vi "test3.vi"() -> ()   [LabVIEW 2020]
uses:
  <vilib>/Platform/TimedLoop/XDataNode/timing_clust.ctl
  <vilib>/Platform/TimedLoop/XDataNode/nitl_modes.ctl
  <vilib>/Platform/TimedLoop/XDataNode/wakeup.ctl
  37583fcc-cec8-480d-a6d0-1da09da3d0dd.vi
  <vilib>/platform/TimedLoop/XDataNode/XDataNode.xnode
  <vilib>/Platform/TimedLoop/XDataNode/XDNodeRunTimeDep.lvlib
panel:
  out "Tank":dbl(slide) scale=0.0..1.0
  out "Current XY":cluster{"X":dbl, "Y":dbl}
  out "XY Graph":cluster{dbl[], dbl[]}[](graph)
  out "Move Time":u32
  out "Distance":dbl
  out "Start Time":u32
  out "Start XY":cluster{"X":dbl, "Y":dbl}
  out "Target XY":cluster{"X":dbl, "Y":dbl}
  out "Stopped":bool
  in  "Stop":bool
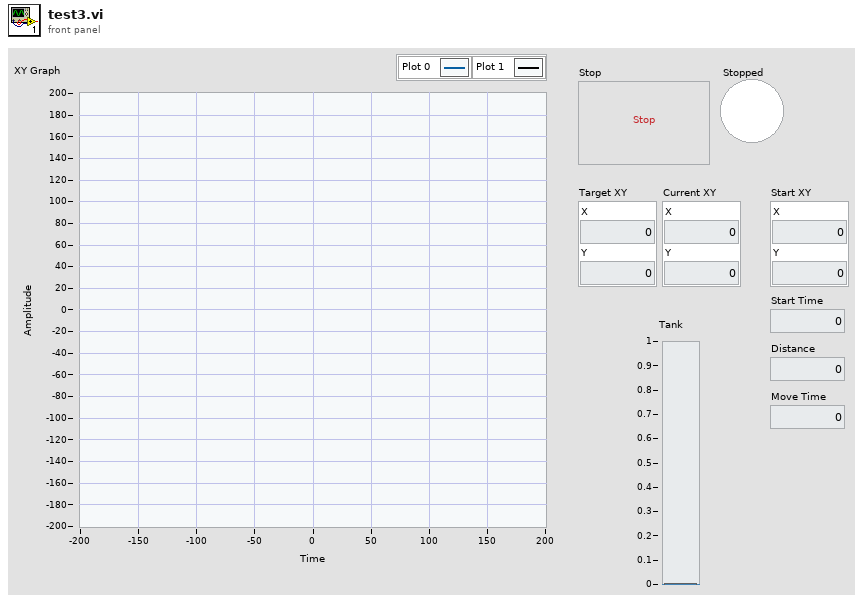
[diagram p1: front panel]
types:
  T1 = typedef "XDNodeRunTimeDep.lvlib/timing_clust.ctl" = cluster{"Expected End [f-1]":u64, "Actual End [f-1]":u64, "Finished Late? [f-1]":bool, "Expected End [i-1]":u64, "Actual End [i-1]":u64, "Finished Late? [i-1]":bool, "Expected Start [i]":u64, "Actual Start [i]":u64, "Expected Start [f]":u64, "Actual Start [f]":u64, "Source Name":string, "Structure Name":string, "Period":i64, "Deadline":i64, "Offset":i64, "Start":i64, "Priority":i32, "Timeout":i32, "Mode":T2, "Wakeup Reason":T3, "Error":errorcluster, "Source Type":string, "Secondary Source Type":string, "Global End Time":u64, "Global Start Time":u64, "Frame Duration":u64, "Iteration Duration":u64, "Assigned CPU":i32, "I/O Scan Engine Mode":u32}
  T2 = typedef "XDNodeRunTimeDep.lvlib/nitl_modes.ctl" = enum32{"No Change", "Process missed periods, maintain original phase", "Discard missed periods, maintain original phase", "Process missed periods, ignore original phase", "Discard missed periods, ignore original phase"}
  T3 = typedef "XDNodeRunTimeDep.lvlib/wakeup.ctl" = enum32{"Normal", "Aborted", "Asynchronous wakeup", "Timing source error", "Timed loop error", "Timeout"}
  T4 = typedef "LVPoint32TypeDef.ctl" = cluster{"Horizontal":i32, "Vertical":i32}
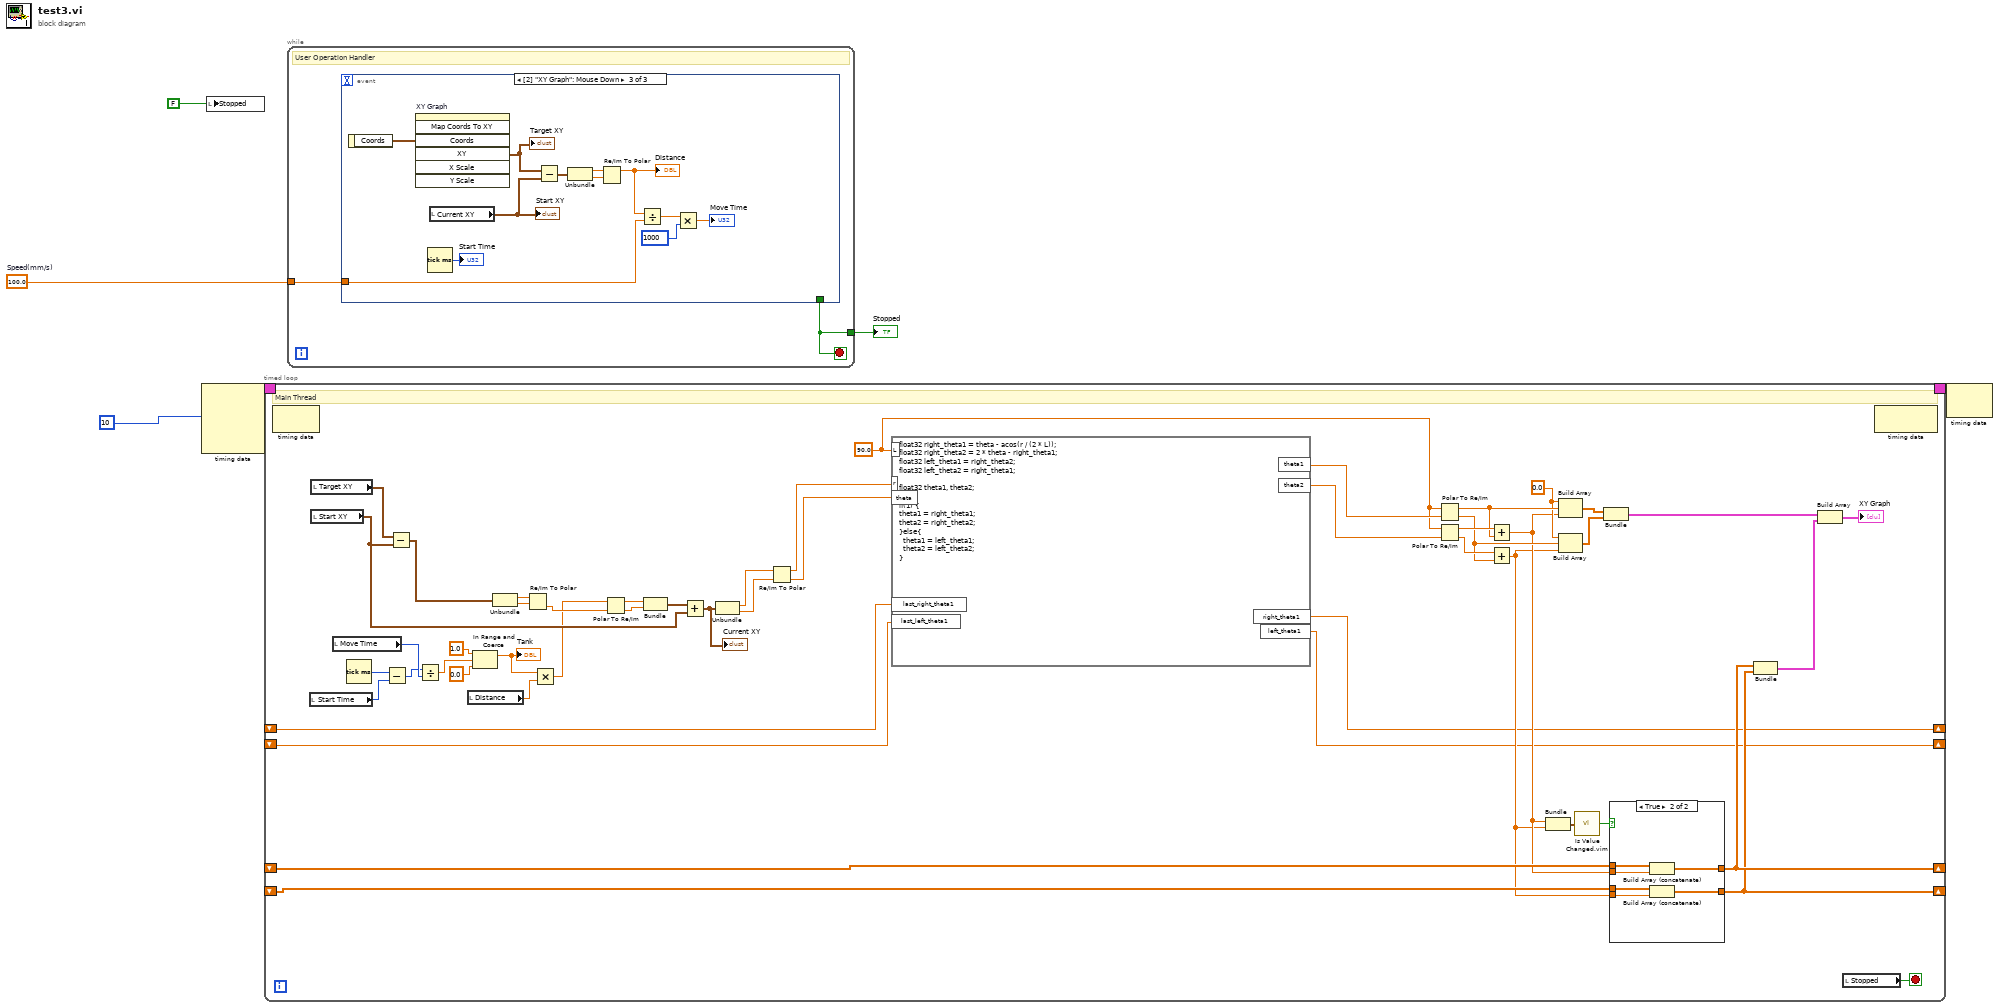
[diagram p0: block diagram]
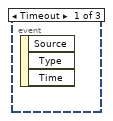
[diagram p3: hidden frame]
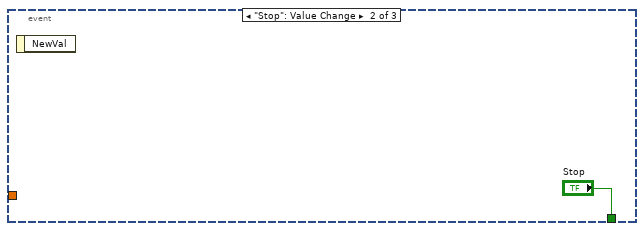
[diagram p4: hidden frame]
diagram:
  w1 = 100.0  # Speed(mm/s)
  n1 = node-c288(i64 10 ("Period")) -> (w6:T1)  [unwired: 3 in]
  n2 = local write "Stopped"(FALSE ("Stopped")) -> ()
  n3 = timed-loop {
    timing: w6 -> [_]
    timing-out: [_] -> w5
    shift-right: [w19] -> _
    shift-left: _ -> [w26]
    shift-right: [w18] -> _
    shift-left: _ -> [w25]
    shift-right: [w9] -> _
    shift-left: _ -> [w8]
    shift-right: [w10] -> _
    shift-left: _ -> [w7]
    stop <- w56 stop-if-true
    w31 = 0.0 ("element")
    w28 = 90.0 ("input variable")
    # "Main Thread"
    n4 = node-c288() -> ()  [unwired: 1 in, 1 out]
    n5 = local read "Start Time"() -> (w54:u32)
    n6 = local read "Target XY"() -> (w53:cluster{"X":dbl, "Y":dbl})
    n7 = local read "Start XY"() -> (w44:cluster{"X":dbl, "Y":dbl})
    n8 = local read "Move Time"() -> (w40:u32)
    n9 = Tick Count (ms)() -> (millisecond timer value=w55:u32)
    n10 = Subtract(x=w55, y=w54) -> (x-y=w15:u32)
    n11 = Subtract(x=w53, y=w44) -> (x-y=w51:cluster{"X":dbl, "Y":dbl})
    n12 = Divide(x=w15, y=w40) -> (x/y=w14:dbl)
    n13 = local read "Distance"() -> (w52:dbl)
    n14 = In Range and Coerce(upper limit=1.0 ("lower limit"), x=w14, lower limit=0.0) -> (coerced(x)=w11:dbl)  [unwired: 1 out]
    "Tank" <- w11
    n15 = Unbundle(w51) -> ("X"=w50:dbl, "Y"=w49:dbl)
    n16 = Re/Im To Polar(2:w49, 3:w50) -> (0:w48:dbl)  [unwired: 1 out]
    n17 = Multiply(x=w11, y=w52) -> (x*y=w39:dbl)
    n18 = Polar To Re/Im(2:w48, 3:w39) -> (0:w46:dbl, 1:w47:dbl)
    n19 = Bundle(w47, w46) -> (w45:cluster{dbl, dbl})  [unwired: 1 in]
    n20 = Add(x=w45, y=w44) -> (x+y=w27:cluster{dbl, dbl})
    "Current XY" <- w27
    n21 = Unbundle(w27) -> (w43:dbl, w42:dbl)
    n22 = Re/Im To Polar(2:w42, 3:w43) -> (0:w41:dbl, 1:w38:dbl)
    n23 = formula code="float32 right_theta1 = theta - acos(r / (2 * L));\nfloat32 right_theta2 = 2 * theta - right_theta1;\nfloat32 left_theta1 = right_theta2;\nfloat32 left_theta2 = right_theta1;\n\nfloat32 theta1, theta2;\n\nif(1) {\ntheta1 = right_theta1;\ntheta2 = right_theta2;\n}else{\n  theta1 = left_theta1;\n  theta2 = left_theta2;\n}"("r"=w38, "theta"=w41, "L"=w28, "last_right_theta1"=w8, "last_left_theta1"=w7) -> ("theta1"=w30:sgl, "theta2"=w29:sgl, "right_theta1"=w9:sgl, "left_theta1"=w10:sgl)
    n24 = Polar To Re/Im(2:w30, 3:w28) -> (0:w34:dbl, 1:w35:dbl)
    n25 = Polar To Re/Im(2:w29, 3:w28) -> (0:w36:dbl, 1:w37:dbl)
    n26 = Add(x=w37, y=w35) -> (x+y=w24:dbl)
    n27 = Add(x=w36, y=w34) -> (x+y=w23:dbl)
    n28 = Bundle(w24, w23) -> (w22:cluster{dbl, dbl})  [unwired: 1 in]
    n29 = Build Array(w31, w35, w24) -> (w33:dbl[])
    n30 = Build Array(w31, w34, w23) -> (w32:dbl[])
    n31 = call "Is Value Changed.vim"("value"=w22) -> ("changed or first call?"=w21:bool)
    n32 = Bundle(w33, w32) -> (w20:cluster{dbl[], dbl[]})  [unwired: 1 in]
    n33 = case shown="True" w21 {
      tunnel: w24 -> [_ w64]
      tunnel: w23 -> [_ w63]
      tunnel: [w58 w62] -> w19
      tunnel: [w57 w61] -> w18
      tunnel: w26 -> [w58 w60]
      tunnel: w25 -> [w57 w59]
      frame False {
      }
      frame True {
        n34 = Build Array (concatenate)(w60, w64) -> (w62:dbl[])
        n35 = Build Array (concatenate)(w59, w63) -> (w61:dbl[])
      }
    }
    n36 = Bundle(w19, w18) -> (w17:cluster{dbl[], dbl[]})  [unwired: 1 in]
    n37 = Build Array(w20, w17) -> (→"XY Graph":cluster{dbl[], dbl[]}[])
    n38 = local read "Stopped"() -> (w56:bool)
    n39 = node-c288() -> ()  [unwired: 1 in, 1 out]
  }
  n40 = while {
    tunnel: [w68] -> w4
    tunnel: w1 -> [w67]
    stop <- w68 stop-if-true
    # "User Operation Handler"
    n41 = event shown="[2] \"XY Graph\": Mouse Down" {
      selector: _ -> [_ _ _]
      dyn-events: _ -> [_ _ _]
      timeout: _ -> [_ _ _]
      tunnel: [_ "Stop" _] -> w68
      tunnel: w67 -> [_ _ w79]
      event Timeout {
        n42 = event-data() -> ()  [unwired: 1 in, 3 out]
      }
      event "Stop": Value Change {
        n43 = event-data() -> ()  [unwired: 1 in, 1 out]
      }
      event "XY Graph": Mouse Down {
        n44 = event-data() -> ("Coords"=w75:T4)  [unwired: 1 in]
        n45 = invoke on="XY Graph" class="XYGraph (strict)" method="Map Coords To XY"("Coords"=w75) -> ("XY"=w74:cluster{"X":dbl, "Y":dbl})  [unwired: 6 in, 6 out]
        "Target XY" <- w74
        n46 = Tick Count (ms)() -> (millisecond timer value=→"Start Time":u32)
        n47 = local read "Current XY"() -> (w73:cluster{"X":dbl, "Y":dbl})
        "Start XY" <- w73
        n48 = Subtract(x=w74, y=w73) -> (x-y=w72:cluster{"X":dbl, "Y":dbl})
        n49 = Unbundle(w72) -> ("X"=w71:dbl, "Y"=w70:dbl)
        n50 = Re/Im To Polar(2:w70, 3:w71) -> (1:w80:dbl)  [unwired: 1 out]
        "Distance" <- w80
        n51 = Divide(x=w80, y=w79) -> (x/y=w78:dbl)
        n52 = Multiply(x=w78, y=u32 1000 ("millisecond timer value")) -> (x*y=→"Move Time":dbl)
      }
    }
  }
  "Stopped" <- w4
  n53 = node-c288(w5) -> ()  [unwired: 1 out]
